vi "Write circulationVelocity.vi"(8 "error in (no error)":errorcluster, 10 "circulationVelocity":dbl, 11 "CirculateSkill in":refnum<class "CirculateSkill.lvclass">) -> (0 "error out":errorcluster, 3 "CirculateSkill out":refnum<class "CirculateSkill.lvclass">)   [LabVIEW 2023]
uses:
  CirculateSkill.lvclass
  C:/Users/ebert/Documents/codes/SSL/repo/SSL_AI/GoToSkill_class/GoToSkill.lvclass
  C:/Users/ebert/Documents/codes/SSL/repo/SSL_AI/Skill_class/Skill.lvclass
  C:/Users/ebert/Documents/codes/SSL/repo/SSL_AI/Circulate_class/CirculateSkill.lvclass
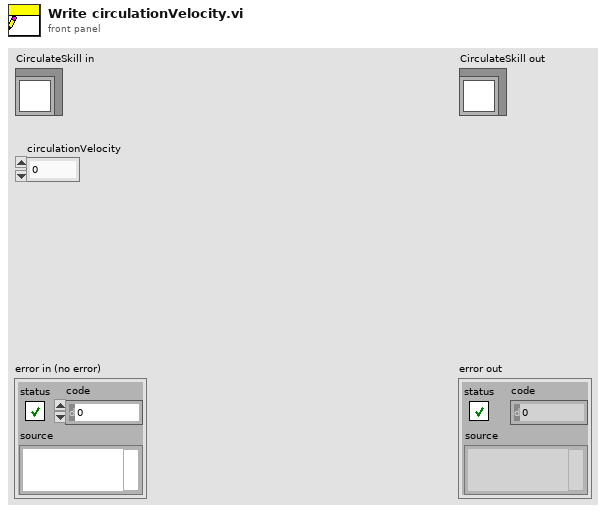
[diagram p1: front panel]
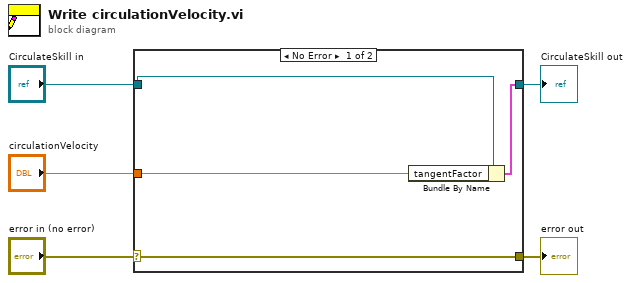
[diagram p0: block diagram]
diagram:
  n1 = case shown="No Error" "error in (no error)" {
    selector: "error in (no error)" -> [w9 w10]
    tunnel: [w9 w10] -> w4
    tunnel: [w7 w11] -> w2
    tunnel: "CirculateSkill in" -> [w8 w11]
    tunnel: "circulationVelocity" -> [w6 _]
    frame No Error {
      n2 = Bundle By Name(cluster=w8, "tangentFactor"=w6) -> (w7:cluster{})
    }
    frame Error {
    }
  }
  "error out" <- w4
  "CirculateSkill out" <- w2
